vi "ANN_VirtualVehiclePosture.vi"(7 "reset":bool, 8 "dt":dbl, 9 "linear velocity":dbl, 11 "trajectory":T2) -> (0 "angular velocity":dbl, 1 "velocity":dbl, 3 "virtual posture":T1)   [LabVIEW 2017]
doc: "This VI returns the reference postures (x, y, O) required to travel <b>trajectory</b>. You can view the execution of this VI as representing a virtual vehicle travelling the <b>trajectory</b> at a velocity of <b>linearV</b>."
uses:
  Trajectory.ctl
  VehiclePosture.ctl
panel:
  # "This is a Virtual vehicle  that will be tracked by the real vehicle. This VI calculate current Posture and (V,V) of Virtual Vehicle according to the trajectory."
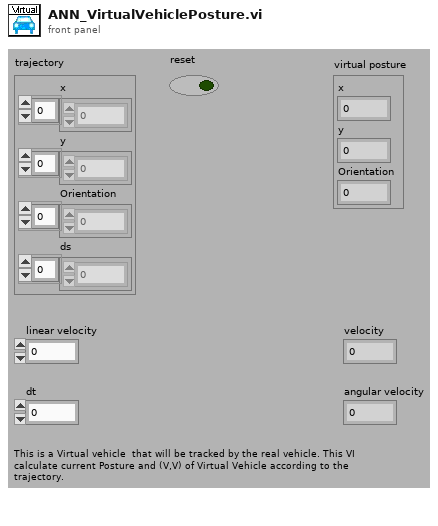
[diagram p1: front panel]
types:
  T1 = typedef "VehiclePosture.ctl" = cluster{"x":dbl, "y":dbl, "Orientation":dbl}
  T2 = typedef "Trajectory.ctl" = cluster{"x":dbl[], "y":dbl[], "Orientation":dbl[], "ds":dbl[]}
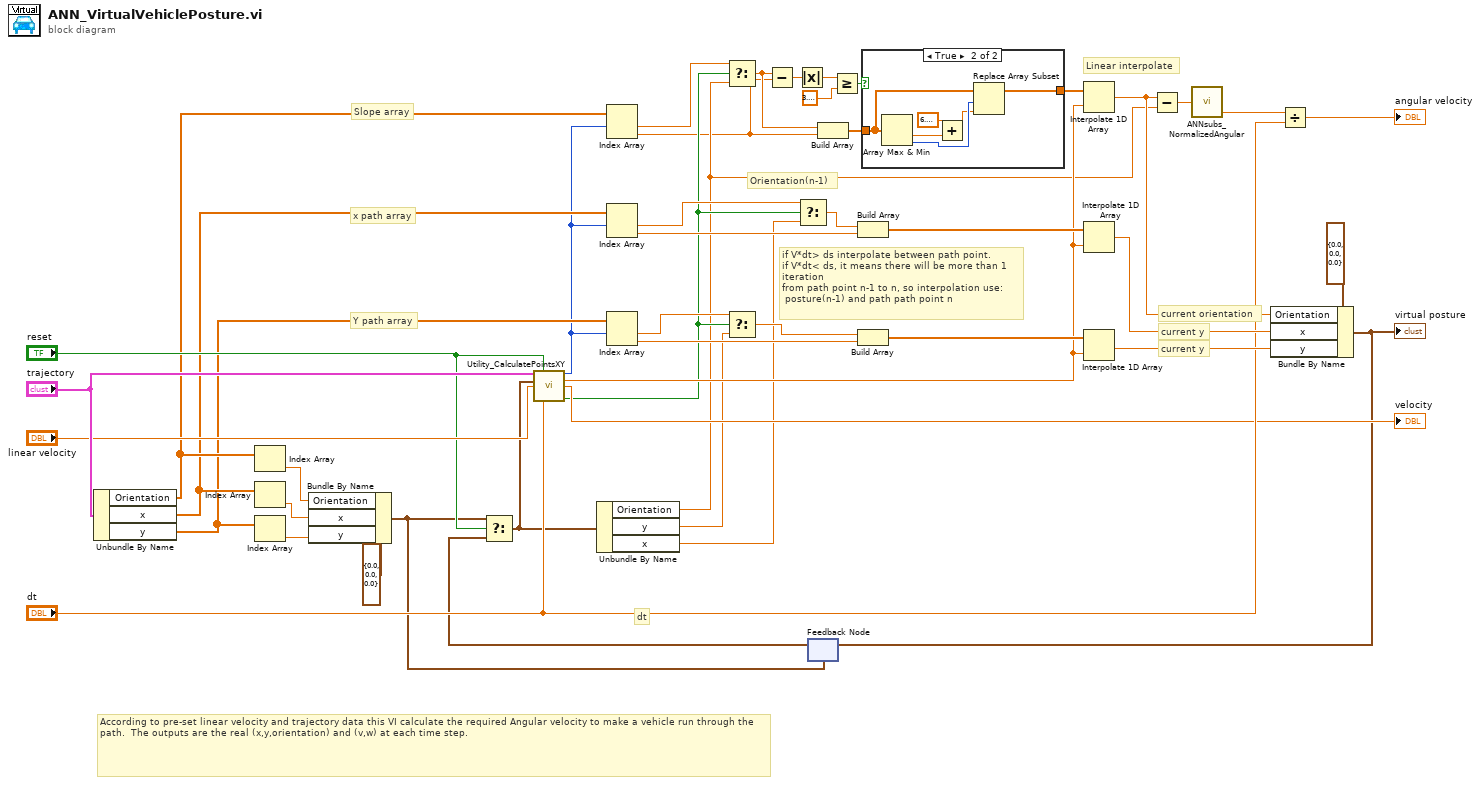
[diagram p0: block diagram]
diagram:
  # "current orientation"
  # "According to pre-set linear velocity and trajectory data this VI calculate the required Angular velocity to make a vehicle run through the path.  The outputs are the real (x,y,orientation) and (v,w) at each time step."
  # "if V*dt> ds interpolate between path point.\nif V*dt< ds, it means there will be more than 1 iteration\nfrom path point n-1 to n, so interpolation use:\n posture(n-1) and path path point n"
  # "Linear interpolate"
  # "current y"
  # "Slope array"
  # "x path array"
  # "Y path array"
  # "dt"
  # "Orientation(n-1)"
  # "current y"
  n1 = Unbundle By Name("trajectory") -> ("Orientation"=w11:dbl[], "x"=w8:dbl[], "y"=w6:dbl[])
  n2 = Index Array(array=w11) -> (element=w9:dbl)  [unwired: 1 in]
  n3 = Index Array(array=w8) -> (element=w7:dbl)  [unwired: 1 in]
  n4 = Index Array(array=w6) -> (element=w5:dbl)  [unwired: 1 in]
  n5 = Bundle By Name(cluster=T1 {"x"=0.0, "y"=0.0, "Orientation"=0.0} ("VehiclePosture"), "Orientation"=w9, "x"=w7, "y"=w5) -> (w1:T1)
  n6 = feedback #1(w1) -> (w12:T1)
  n7 = Select(t=w1, s="reset", f=w12) -> (s? t:f=w13:T1)
  n8 = call "Utility_CalculatePointsXY.vi"("trajectory"="trajectory", "reset"="reset", "Posture(n-1)"=w13, "linearV"="linear velocity", "dt"="dt") -> ("index"=w4:i32, "fractional index"=w19:dbl, "desired LinearV"=→"velocity":dbl, "cross 2 elements"=w18:bool)  [unwired: 7 in]
  n9 = Unbundle By Name(w13) -> ("Orientation"=w15:dbl, "y"=w17:dbl, "x"=w16:dbl)
  n10 = Index Array(array=w11, index #1=w4) -> (element #1=w3:dbl, element #2=w2:dbl)  [unwired: 1 in]
  n11 = Index Array(array=w8, index #1=w4) -> (element #1=w25:dbl, element #2=w29:dbl)  [unwired: 1 in]
  n12 = Index Array(array=w6, index #1=w4) -> (element #1=w26:dbl, element #2=w46:dbl)  [unwired: 1 in]
  n13 = Select(t=w3, s=w18, f=w15) -> (s? t:f=w27:dbl)
  n14 = Select(t=w26, s=w18, f=w17) -> (s? t:f=w30:dbl)
  n15 = Subtract(x=w27, y=w2) -> (x-y=w43:dbl)
  n16 = Absolute Value(x=w43) -> (abs(x)=w42:dbl)
  n17 = Select(t=w25, s=w18, f=w16) -> (s? t:f=w28:dbl)
  n18 = Build Array(w27, w2) -> (w39:dbl[])
  n19 = Greater Or Equal?(x=w42, y=3.141592653589793) -> (x >= y?=w40:bool)
  n20 = Build Array(w28, w29) -> (w44:dbl[])
  n21 = Build Array(w30, w46) -> (w45:dbl[])
  n22 = case shown="True" w40 {
    tunnel: w39 -> [w47 w51]
    tunnel: [w47 w48] -> w38
    frame False {
    }
    frame True {
      n23 = Array Max & Min(array=w51) -> (min value=w53:dbl, min index (indices)=w50:i32)  [unwired: 2 out]
      n24 = Add(x=6.283185307179586, y=w53) -> (x+y=w49:dbl)
      n25 = Replace Array Subset(array=w51, new element=w49, index=w50) -> (w48:dbl[])
    }
  }
  n26 = Interpolate 1D Array(1:w19, 2:w38) -> (0:w33:dbl)
  n27 = Interpolate 1D Array(1:w19, 2:w44) -> (0:w32:dbl)
  n28 = Interpolate 1D Array(1:w19, 2:w45) -> (0:w31:dbl)
  n29 = Subtract(x=w33, y=w15) -> (x-y=w37:dbl)
  n30 = call "ANNsubs_NormalizedAngular.vi"("Delta angle"=w37) -> ("Delta angle out"=w36:dbl)
  n31 = Bundle By Name(cluster=T1 {"x"=0.0, "y"=0.0, "Orientation"=0.0} ("VehiclePosture"), "Orientation"=w33, "x"=w32, "y"=w31) -> (w20:T1)
  "virtual posture" <- w20
  n32 = feedback-in #1(w20) -> ()
  n33 = Divide(x=w36, y="dt") -> (x/y=→"angular velocity":dbl)
